vi "Release Queues.vi"(8 "error in (no error)":errorcluster, 9 "Q3":refnum<queue>, 10 "Q2 Cluster":T1, 11 "Q1":refnum<queue>) -> (0 "error out":errorcluster)   [LabVIEW 2014]
doc: "<B>Copyright</B>: (c) MHWirth 2015. All rights reserved.\n\nThis subVI releases queues that are used for this application at the end of operation."
uses:
  TypeDef/Q1 Message.ctl
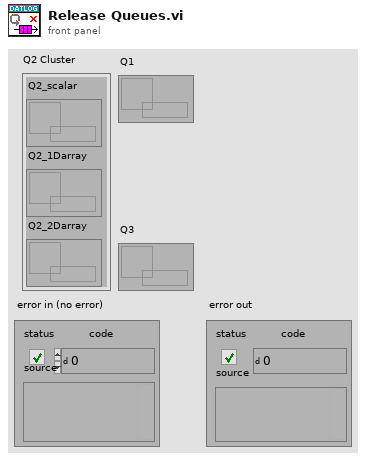
[diagram p1: front panel]
types:
  T1 = cluster{"Q2_scalar":refnum<queue>, "Q2_1Darray":refnum<queue>, "Q2_2Darray":refnum<queue>}
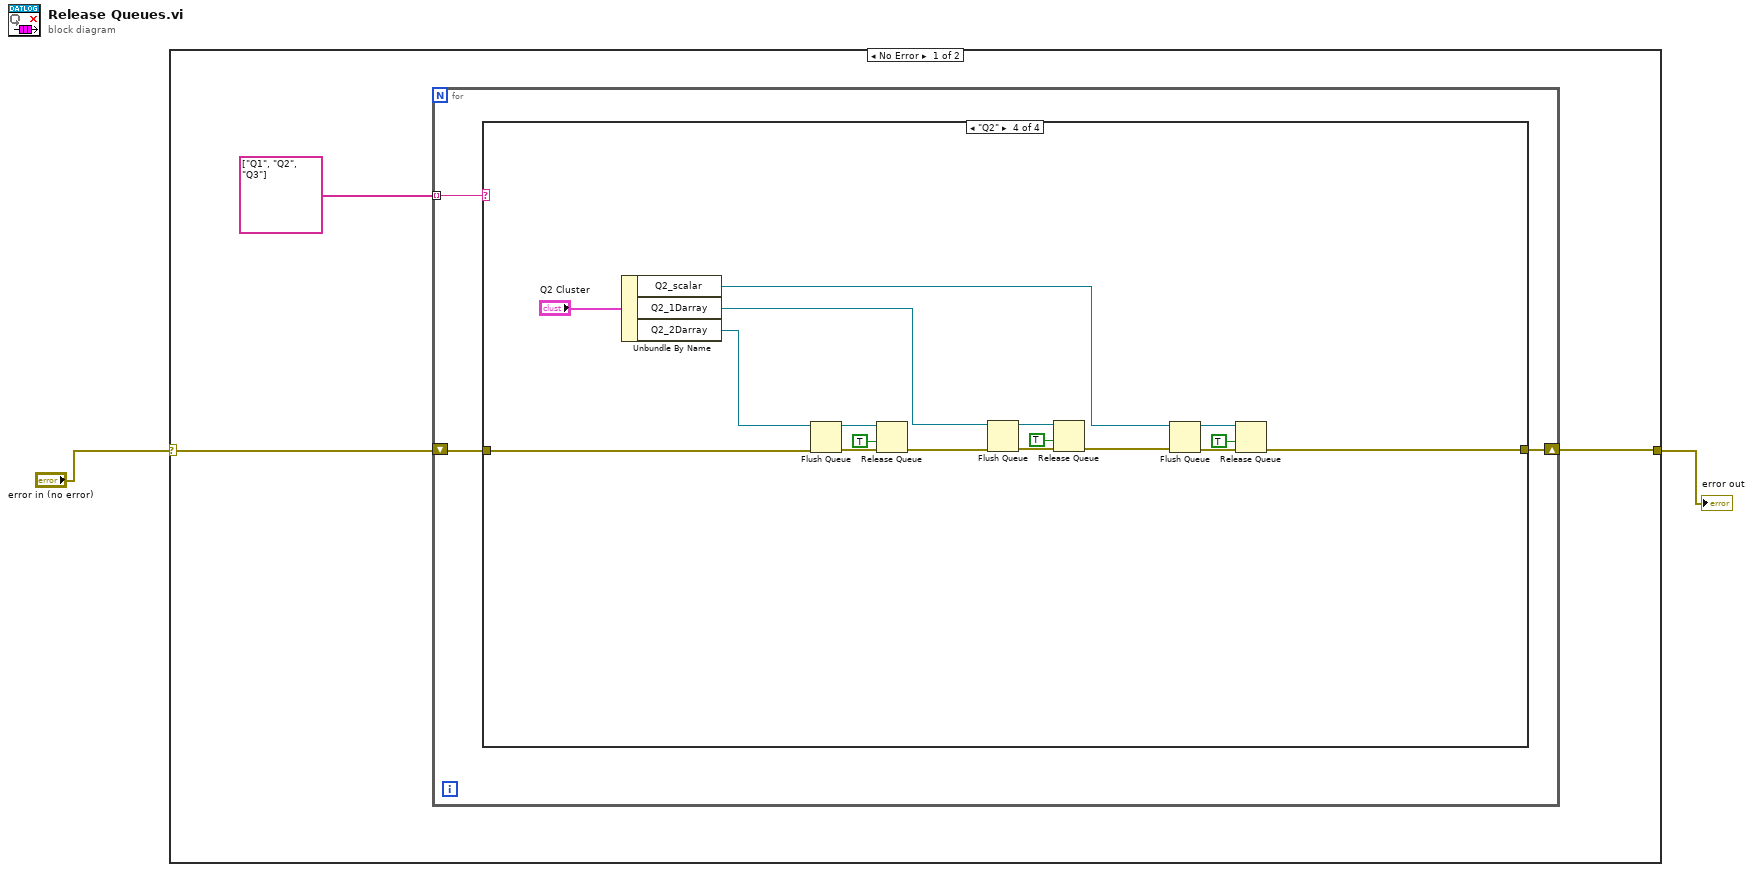
[diagram p0: block diagram]
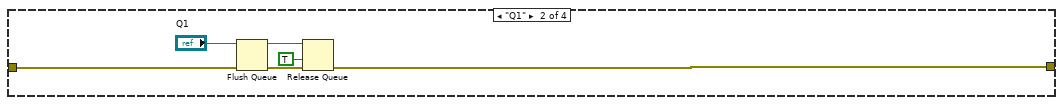
[diagram p3: hidden frame]
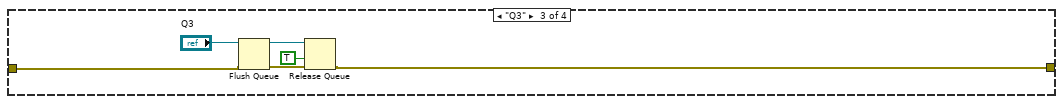
[diagram p4: hidden frame]
diagram:
  n1 = case shown="No Error" "error in (no error)" {
    selector: "error in (no error)" -> [w4 w39]
    tunnel: [w3 w39] -> w1
    frame No Error {
      n2 = for {
        tunnel: string[] ["Q1", "Q2", "Q3"] -> [w8] mode=indexing
        shift-right: [w6] -> w3
        shift-left: w4 -> [w7]
        n3 = case shown="\"Q2\"" w8 {
          tunnel: w7 -> [w9 w14 w18 w28]
          tunnel: [w9 w12 w17 w25] -> w6
          frame "do nothing", Default {
          }
          frame "Q1" {
            n4 = Flush Queue(queue="Q1", error in (no error)=w14) -> (queue out=w11:refnum<queue>, error out=w13:errorcluster)  [unwired: 1 out]
            n5 = Release Queue(queue=w11, force destroy? (F)=TRUE, error in (no error)=w13) -> (error out=w12:errorcluster)  [unwired: 2 out]
          }
          frame "Q3" {
            n6 = Flush Queue(queue="Q3", error in (no error)=w18) -> (queue out=w20:refnum<queue>, error out=w21:errorcluster)  [unwired: 1 out]
            n7 = Release Queue(queue=w20, force destroy? (F)=TRUE, error in (no error)=w21) -> (error out=w17:errorcluster)  [unwired: 2 out]
          }
          frame "Q2" {
            n8 = Unbundle By Name("Q2 Cluster") -> ("Q2_scalar"=w22:refnum<queue>, "Q2_1Darray"=w23:refnum<queue>, "Q2_2Darray"=w24:refnum<queue>)
            n9 = Flush Queue(queue=w24, error in (no error)=w28) -> (queue out=w36:refnum<queue>, error out=w37:errorcluster)  [unwired: 1 out]
            n10 = Release Queue(queue=w36, force destroy? (F)=TRUE, error in (no error)=w37) -> (error out=w27:errorcluster)  [unwired: 2 out]
            n11 = Flush Queue(queue=w23, error in (no error)=w27) -> (queue out=w33:refnum<queue>, error out=w32:errorcluster)  [unwired: 1 out]
            n12 = Release Queue(queue=w33, force destroy? (F)=TRUE, error in (no error)=w32) -> (error out=w26:errorcluster)  [unwired: 2 out]
            n13 = Flush Queue(queue=w22, error in (no error)=w26) -> (queue out=w30:refnum<queue>, error out=w31:errorcluster)  [unwired: 1 out]
            n14 = Release Queue(queue=w30, force destroy? (F)=TRUE, error in (no error)=w31) -> (error out=w25:errorcluster)  [unwired: 2 out]
          }
        }
      }
    }
    frame Error {
    }
  }
  "error out" <- w1
